vi "Begin (Mark Siekmeier's conflicted copy 2013-04-30).vi"(11 "Image Size":T1=enum."160x120") -> (0 "error out":errorcluster)   [LabVIEW 2012]
doc: "Called before other user functions, this VI is expected to open initial I/O refnums, load in file data, and do all program initialization. Notice that the <B>error out</B> terminal is simply used for data flow. Wiring it to other structures or subVIs ensures that this VI runs first."
uses:
  <vilib>/Rock Robotics/WPI/Camera/WPI_CameraImageSize.ctl
  <vilib>/Rock Robotics/WPI/Camera/WPI_CameraWhite Balance Values.ctl
  <vilib>/Rock Robotics/WPI/Camera/WPI_CameraExposure Values.ctl
  <vilib>/Rock Robotics/WPI/Camera/WPI_CameraFrameRate.ctl
  <vilib>/Rock Robotics/WPI/DriverStation/WPI_DriverStationRobotMode2.ctl
  <vilib>/Rock Robotics/WPI/Joystick/WPI_JoystickDeviceEnum.ctl
  <vilib>/Rock Robotics/SystemInterfaces/Typedef/FPGA_TypedefDigitalModule.ctl
  <vilib>/Rock Robotics/SystemInterfaces/DIO/FPGA_DIOPWMChannel.ctl
  <vilib>/Rock Robotics/WPI/Solenoid/WPI_SolenoidChannel.ctl
  <vilib>/Rock Robotics/SystemInterfaces/Typedef/FPGA_TypedefSolenoidModule.ctl
  <vilib>/Rock Robotics/WPI/Solenoid/WPI_SolenoidValue.ctl
  <vilib>/Rock Robotics/SystemInterfaces/DIO/FPGA_DIOChannel.ctl
  <vilib>/Rock Robotics/WPI/Encoder/WPI_EncoderType.ctl
  <vilib>/Rock Robotics/WPI/SafetyOutput/WPI_SafetyOutputConfigMenu.ctl
  <vilib>/Rock Robotics/SystemInterfaces/DIO/FPGA_DIORelayChannel.ctl
  <vilib>/Rock Robotics/SystemInterfaces/Typedef/FPGA_TypedefAnalogModuleForGyro.ctl
  <vilib>/Rock Robotics/SystemInterfaces/AI/FPGA_AIGyroChannel.ctl
  Robot Global Data.vi
  <vilib>/Rock Robotics/WPI/Solenoid/WPI_SolenoidOpenSingle.vi
  <vilib>/Rock Robotics/WPI/Solenoid/WPI_SolenoidSetEnum.vi
  <vilib>/Rock Robotics/WPI/Counter/WPI_CounterDigitalInputToDigitalSource.vi
  <vilib>/Rock Robotics/WPI/RobotDrive/WPI_RobotDriveOpen2MotorWithTalon.vi
  <vilib>/Rock Robotics/WPI/Solenoid/WPI_SolenoidOpenDouble.vi
  <vilib>/Rock Robotics/WPI/MotorControl/WPI_MotorControlOpen Talon.vi
  <vilib>/Rock Robotics/WPI/Compressor/WPI_CompressorGetSetRefNum.vi
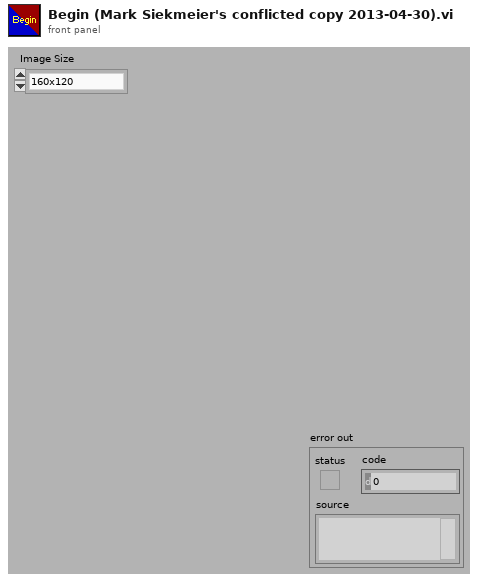
[diagram p1: front panel]
types:
  T1 = typedef "WPI_CameraImageSize.ctl" = enum16{"640x480", "320x240", "160x120"}
  T2 = typedef "FPGA_AIGyroChannel.ctl" = enum8{"AI 1", "AI 2", "Invalid"}
  T3 = typedef "FPGA_TypedefAnalogModuleForGyro.ctl" = enum16{"Analog Module 1"}
  T4 = typedef "WPI_SolenoidChannel.ctl" = enum8{"Solenoid 1", "Solenoid 2", "Solenoid 3", "Solenoid 4", "Solenoid 5", "Solenoid 6", "Solenoid 7", "Solenoid 8", "Invalid"}
  T5 = typedef "WPI_SolenoidValue.ctl" = enum16{"Off", "On", "Forward", "Reverse"}
  T6 = typedef "FPGA_DIOChannel.ctl" = enum8{"DIO 1", "DIO 2", "DIO 3", "DIO 4", "DIO 5", "DIO 6", "DIO 7", "DIO 8", "DIO 9", "DIO 10", "DIO 11", "DIO 12", "DIO 13", "DIO 14", "Invalid"}
  T7 = typedef "FPGA_DIORelayChannel.ctl" = enum8{"Relay 1", "Relay 2", "Relay 3", "Relay 4", "Relay 5", "Relay 6", "Relay 7", "Relay 8", "Invalid"}
  T8 = typedef "FPGA_TypedefDigitalModule.ctl" = enum16{"Digital Module 1", "Digital Module 2"}
  T9 = typedef "WPI_SafetyOutputConfigMenu.ctl" = enum16{"Enable", "Disable"}
  T10 = typedef "FPGA_DIOPWMChannel.ctl" = enum8{"PWM 1", "PWM 2", "PWM 3", "PWM 4", "PWM 5", "PWM 6", "PWM 7", "PWM 8", "PWM 9", "PWM 10", "Invalid"}
  T11 = typedef "WPI_EncoderType.ctl" = enum16{"1x", "2x", "4x"}
  T12 = typedef "FPGA_TypedefSolenoidModule.ctl" = enum16{"Solenoid Module 1", "Solenoid Module 2"}
  T13 = typedef "WPI_JoystickDeviceEnum.ctl" = enum16{"USB 1", "USB 2", "USB 3", "USB 4", "Kinect 1", "Kinect 2"}
  T14 = typedef "WPI_DriverStationRobotMode2.ctl" = enum16{"Autonomous Disabled", "Autonomous Enabled", "Teleop Disabled", "Teleop Enabled", "Timeout", "Finish", "Test Disabled", "Test Enabled"}
  T15 = typedef "WPI_CameraFrameRate.ctl" = u32
  T16 = typedef "WPI_CameraExposure Values.ctl" = enum16{"Auto", "Flicker-free 50 Hz", "Flicker-free 60 Hz", "Hold current"}
  T17 = typedef "WPI_CameraWhite Balance Values.ctl" = enum16{"Auto", "Fixed indoor", "Fixed outdoor 1", "Fixed outdoor 2", "Fixed fluorescent 1", "Fixed fluorescent 2", "Hold current"}
  T18 = typedef "WPI_DigitalInputDevRef.ctl" = cluster{"DevStatus":errorcluster, "DIO Channel":T6, "Digital Module":T8}
  T19 = typedef "WPI_CompressorDevRef.ctl" = cluster{"DevStatus":errorcluster, "DigitalInputDevRef":T18, "RelayDevRef":T20}
  T20 = typedef "WPI_RelayDevRef.ctl" = cluster{"DevStatus":errorcluster, "Relay Channel":T7, "Digital Module":T8, "Relay Direction":T21}
  T21 = typedef "WPI_RelayDirection.ctl" = enum16{"Both directions", "Forward only", "Reverse only"}
  T22 = typedef "FPGA_CounterEncoderSourceConvertionLVSourceType.ctl" = cluster{"DevStatus":errorcluster, "AnalogTriggerMode?":bool, "DigitalMode":cluster{"Digital Module":T8, "DIO Channel":T23}, "AnalogTriggerMode":cluster{"AnalogTriggerIndex":T24, "OutputType":T25}}
  T23 = typedef "FPGA_DIODigitalSourceChannel.ctl" = enum8{"DIO 1", "DIO 2", "DIO 3", "DIO 4", "DIO 5", "DIO 6", "DIO 7", "DIO 8", "DIO 9", "DIO 10", "DIO 11", "DIO 12", "DIO 13", "DIO 14", "Disabled"}
  T24 = typedef "FPGA_AnalogTriggerIndex.ctl" = enum8{"Trig 0", "Trig 1", "Trig 2", "Trig 3", "Trig 4", "Trig 5", "Trig 6", "Trig 7", "Invalid"}
  T25 = typedef "FPGA_AnalogTriggerOutType.ctl" = enum16{"InWindow", "TriggerState", "Rising", "Falling"}
  T26 = typedef "WPI_JoystickDevRef.ctl" = cluster{"Device":T13}
  T27 = typedef "WPI_CameraDevRef.ctl" = cluster{"Camera Address":string, "CameraStatus":errorcluster, "Acquire Image Notifier":refnum<notifier>}
  T28 = typedef "WPI_RobotDriveDevRef.ctl" = cluster{"DevStatus":errorcluster, "Motors[]":T29[], "Square Inputs":bool, "Max Output":dbl, "Isochronous":bool}
  T29 = typedef "WPI_MotorControlDeviceRef.ctl" = cluster{"DeviceStatus":errorcluster, "Type":enum16{"PWM", "CAN"}, "PWM":cluster{"Digital Module":T8, "PWM Channel":T10, "DeadBand":T30}, "CAN":cluster{"Device Number":u8, "Control Mode":T31, "Semaphore":T32, "Max Vout":dbl}, "Invert":bool, "TransformRef":T33, "InvTransformRef":T33}
  T30 = typedef "WPI_PWMDeadband.ctl" = cluster{"Name":string, "maxPositivePwm":i32, "minPositivePwm":i32, "centerPwm":i32, "maxNegativePwm":i32, "minNegativePwm":i32, "angularRange":u16}
  T31 = typedef "WPI_CANJaguar_ControlMode.ctl" = enum8{"Percent VBus", "Current", "Speed", "Position", "Voltage"}
  T32 = typedef "Semaphore RefNum" = refnum<k1>
  T33 = typedef "WPI_PWMTransform_ConPane.ctl" = refnum<vi>
  T34 = typedef "WPI_EncoderDevRef.ctl" = cluster{"DevStatus":errorcluster, "EncoderIndex":T35, "CounterIndex":T36, "DistancePerCount":dbl, "Decoding Type":T11}
  T35 = typedef "FPGA_EncoderIdx.ctl" = enum8{"Enc 0", "Enc 1", "Enc 2", "Enc 3", "Invalid"}
  T36 = typedef "FPGA_CounterCtrSystemIndex.ctl" = enum8{"Ctr 0", "Ctr 1", "Ctr 2", "Ctr 3", "Ctr 4", "Ctr 5", "Ctr 6", "Ctr 7", "Invalid"}
  T37 = typedef "WPI_SolenoidDevRef.ctl" = cluster{"DevStatus":errorcluster, "Solenoid Module":T12, "Forward Solenoid Channel":T4, "Reverse Solenoid Channel":T4}
  T38 = typedef "WPI_GyroDevRef.ctl" = cluster{"DevStatus":errorcluster, "Analog Module":T39, "Analog Channel":T40, "Offset":dbl, "Gain (VoltsPerDegree/Second)":dbl}
  T39 = typedef "FPGA_TypedefAnalogModule.ctl" = enum16{"Analog Module 1", "Analog Module 2"}
  T40 = typedef "FPGA_AIChannel.ctl" = enum8{"AI 1", "AI 2", "AI 3", "AI 4", "AI 5", "AI 6", "AI 7", "AI 8", "Invalid"}
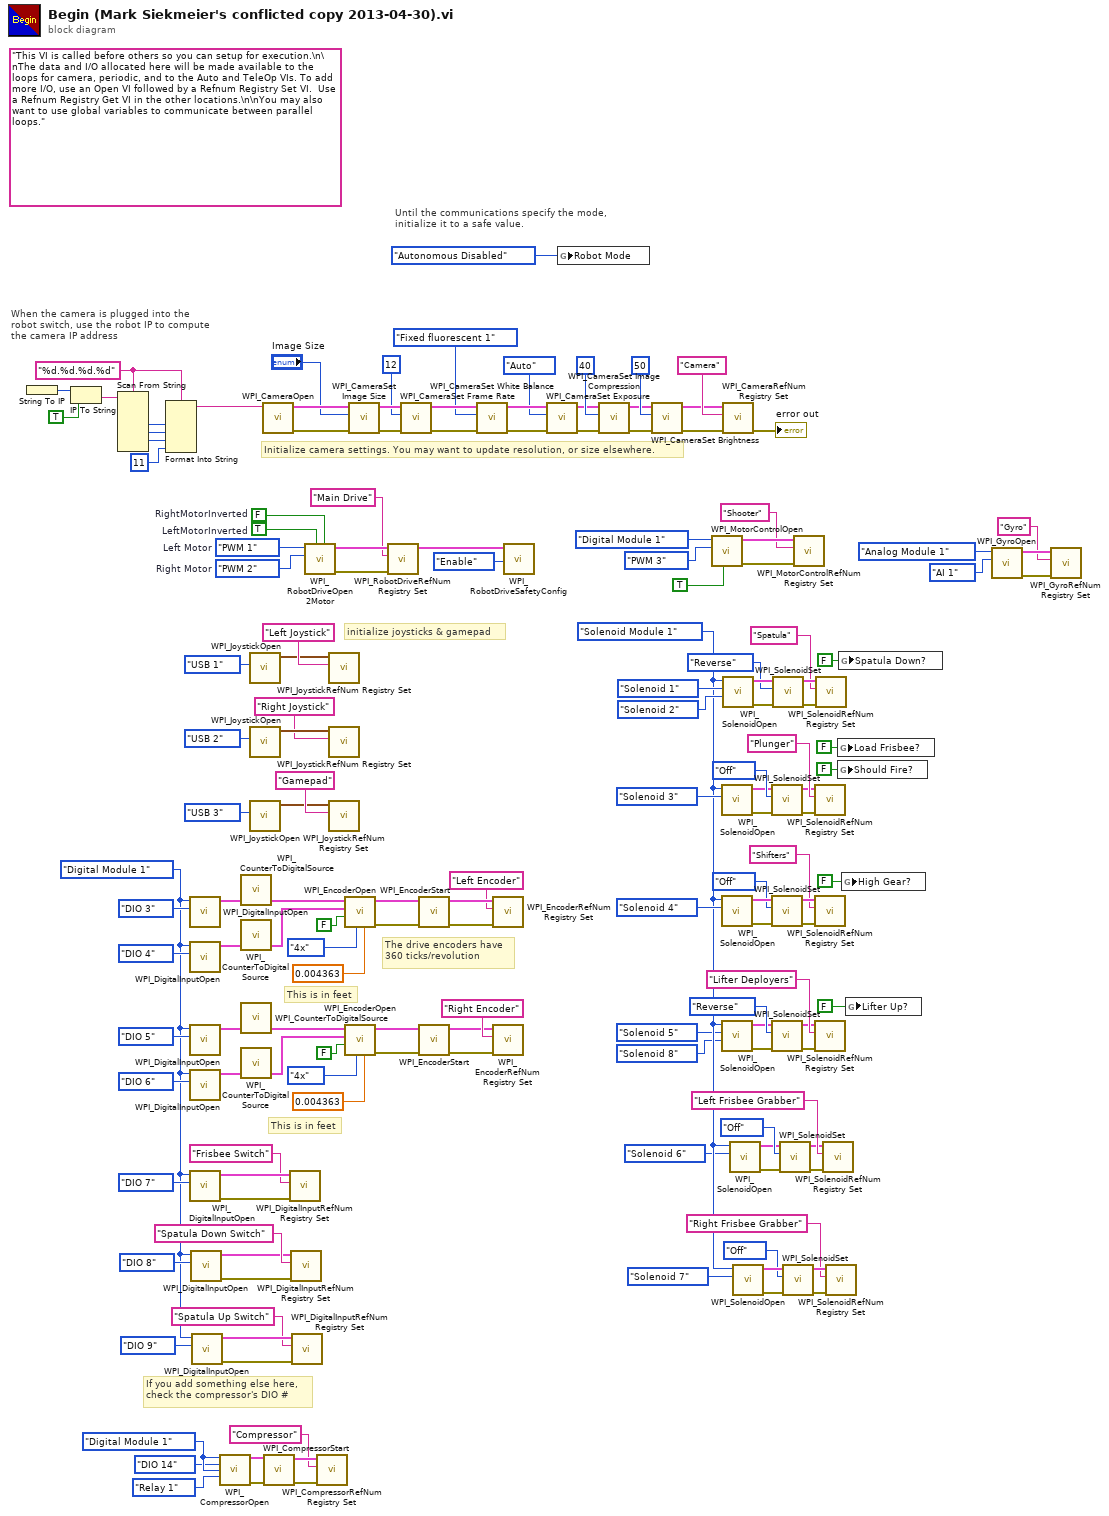
[diagram p0: block diagram]
diagram:
  w47 = FPGA_TypedefDigitalModule."Digital Module 1" ("Pressure Switch Digital Module (Module 1)")
  w65 = FPGA_DIOPWMChannel."PWM 2"  # Right Motor
  w66 = FPGA_DIOPWMChannel."PWM 1"  # Left Motor
  w70 = TRUE  # LeftMotorInverted
  w71 = FALSE  # RightMotorInverted
  w29 = FPGA_TypedefSolenoidModule."Solenoid Module 1" ("Solenoid Module (Module 1)")
  w31 = FPGA_TypedefDigitalModule."Digital Module 1" ("Digital Module (Module 1)")
  w132 = "%d.%d.%d.%d" ("format string")
  (unwired) "This VI is called before others so you can setup for execution.\n\nThe data and I/O allocated here will be made available to the loops for camera, periodic, and to the Auto and TeleOp VIs. To add more I/O, use an Open VI followed by a Refnum Registry Set VI.  Use a Refnum Registry Get VI in the other locations.\n\nYou may also want to use global variables to communicate between parallel loops."
  # "If you add something else here,\ncheck the compressor's DIO #"
  # "The drive encoders have\n360 ticks/revolution"
  # "This is in feet"
  # "This is in feet"
  # "initialize joysticks & gamepad"
  # "Until the communications specify the mode,\ninitialize it to a safe value."
  # "When the camera is plugged into the\nrobot switch, use the robot IP to compute\nthe camera IP address"
  # "Initialize camera settings. You may want to update resolution, or size elsewhere."
  n1 = String To IP() -> (0:w139:u32)  [unwired: 1 in]
  n2 = IP To String(1:TRUE ("dot notation? (F)"), 2:w139) -> (0:w137:string)
  n3 = Scan From String(format string=w132, input string=w137) -> (output 1=w136:i32, output 2=w135:i32, output 3=w134:i32)  [unwired: 7 in, 3 out]
  n4 = Format Into String(format string=w132, w136, w135, w134, 11 ("Compression")) -> (resulting string=w130:string)  [unwired: 2 in, 1 out]
  n5 = call <vilib>:"WPI_DigitalInputOpen.vi"("DIO Channel"=FPGA_DIOChannel."DIO 3" ("CS Channel"), "Digital Module (Module 1)"=w31) -> ("DigitalInputDevRef"=w93:T18)  [unwired: 1 in, 8 out]
  n6 = call <vilib>:"WPI_DigitalInputOpen.vi"("DIO Channel"=FPGA_DIOChannel."DIO 4" ("Clock Channel"), "Digital Module (Module 1)"=w31) -> ("DigitalInputDevRef"=w94:T18)  [unwired: 1 in, 8 out]
  n7 = call <vilib>:"WPI_DigitalInputOpen.vi"("DIO Channel"=FPGA_DIOChannel."DIO 5" ("CS Channel"), "Digital Module (Module 1)"=w31) -> ("DigitalInputDevRef"=w78:T18)  [unwired: 1 in, 8 out]
  n8 = call <vilib>:"WPI_DigitalInputOpen.vi"("DIO Channel"=FPGA_DIOChannel."DIO 6" ("Clock Channel"), "Digital Module (Module 1)"=w31) -> ("DigitalInputDevRef"=w77:T18)  [unwired: 1 in, 8 out]
  n9 = call <vilib>:"WPI_DigitalInputOpen.vi"("DIO Channel"=FPGA_DIOChannel."DIO 7", "Digital Module (Module 1)"=w31) -> ("error out"=w49:errorcluster, "DigitalInputDevRef"=w50:T18)  [unwired: 8 in]
  n10 = call <vilib>:"WPI_DigitalInputOpen.vi"("DIO Channel"=FPGA_DIOChannel."DIO 8", "Digital Module (Module 1)"=w31) -> ("error out"=w38:errorcluster, "DigitalInputDevRef"=w37:T18)  [unwired: 8 in]
  n11 = call <vilib>:"WPI_DigitalInputOpen.vi"("DIO Channel"=FPGA_DIOChannel."DIO 9", "Digital Module (Module 1)"=w31) -> ("error out"=w33:errorcluster, "DigitalInputDevRef"=w34:T18)  [unwired: 8 in]
  n12 = call <vilib>:"WPI_CompressorOpen.vi"("Pressure Switch Digital Module (Module 1)"=w47, "Pressure Switch DIO Channel"=FPGA_DIOChannel."DIO 14", "Relay Digital Module (Module 1)"=w47, "Relay Channel"=FPGA_DIORelayChannel."Relay 1") -> ("CompressorDevRef"=w43:T19, "error out"=w44:errorcluster)  [unwired: 10 in]
  n13 = call-poly <vilib>:"WPI_CounterToDigitalSource.vi"("DigitalInputDevRef"=w93) -> ("Digital Source"=w90:T22)  [unwired: 6 out]
  n14 = call-poly <vilib>:"WPI_CounterToDigitalSource.vi"("DigitalInputDevRef"=w94) -> ("Digital Source"=w91:T22)  [unwired: 6 out]
  n15 = call-poly <vilib>:"WPI_CounterToDigitalSource.vi"("DigitalInputDevRef"=w78) -> ("Digital Source"=w81:T22)  [unwired: 6 out]
  n16 = call-poly <vilib>:"WPI_CounterToDigitalSource.vi"("DigitalInputDevRef"=w77) -> ("Digital Source"=w80:T22)  [unwired: 6 out]
  n17 = call <vilib>:"WPI_JoystickOpen.vi"("JoystickDevice"=WPI_JoystickDeviceEnum."USB 1") -> ("JoystickDevRef"=w128:T26)  [unwired: 10 in]
  n18 = call <vilib>:"WPI_JoystickOpen.vi"("JoystickDevice"=WPI_JoystickDeviceEnum."USB 2") -> ("JoystickDevRef"=w124:T26)  [unwired: 10 in]
  n19 = call <vilib>:"WPI_JoystickOpen.vi"("JoystickDevice"=WPI_JoystickDeviceEnum."USB 3") -> ("JoystickDevRef"=w121:T26)  [unwired: 10 in]
  n20 = call <vilib>:"WPI_CameraOpen.vi"("Camera Address"=w130) -> ("error out"=w151:errorcluster, "CameraDevRef"=w152:T27)  [unwired: 1 in, 8 out]
  n21 = call <vilib>:"WPI_CompressorStart.vi"("error in (no error)"=w44, "CompressorDevRef"=w43) -> ("error out"=w42:errorcluster, "CompressorDevRef"=w41:T19)  [unwired: 8 in]
  n22 = call <vilib>:"WPI_DigitalInputRefNum Registry Set.vi"("error in (no error)"=w49, "refnum name"="Frisbee Switch", "DigitalInputDevRef"=w50) -> ()  [unwired: 7 in, 2 out]
  n23 = call <vilib>:"WPI_DigitalInputRefNum Registry Set.vi"("error in (no error)"=w38, "refnum name"="Spatula Down Switch", "DigitalInputDevRef"=w37) -> ()  [unwired: 7 in, 2 out]
  n24 = call <vilib>:"WPI_DigitalInputRefNum Registry Set.vi"("error in (no error)"=w33, "refnum name"="Spatula Up Switch", "DigitalInputDevRef"=w34) -> ()  [unwired: 7 in, 2 out]
  n25 = call-poly <vilib>:"WPI_RobotDriveOpen2Motor.vi"("Right Motor Inverted"=w71, "Left Motor Inverted"=w70, "Right Motor"=w65, "Left Motor"=w66) -> ("error out"=w67:errorcluster, "RobotDriveDevRef"=w69:T28)  [unwired: 1 in, 5 out]
  n26 = call <vilib>:"WPI_CompressorRefNum Registry Set.vi"("error in (no error)"=w42, "refnum name"="Compressor", "CompressorDevRef"=w41) -> ()  [unwired: 7 in, 2 out]
  n27 = call <vilib>:"WPI_JoystickRefNum Registry Set.vi"("refnum name"="Left Joystick", "JoystickDevRef"=w128) -> ()  [unwired: 8 in, 2 out]
  n28 = call <vilib>:"WPI_JoystickRefNum Registry Set.vi"("refnum name"="Right Joystick", "JoystickDevRef"=w124) -> ()  [unwired: 8 in, 2 out]
  n29 = call <vilib>:"WPI_JoystickRefNum Registry Set.vi"("refnum name"="Gamepad", "JoystickDevRef"=w121) -> ()  [unwired: 8 in, 2 out]
  n30 = call <vilib>:"WPI_EncoderOpen.vi"("DistancePerCount"=0.004363, "Decoding Type"=WPI_EncoderType."4x", "Invert Direction (False)"=FALSE, "BSource"=w91, "ASource"=w90) -> ("error out"=w96:errorcluster, "EncoderDevRef"=w95:T34)  [unwired: 5 in]
  n31 = call <vilib>:"WPI_EncoderOpen.vi"("DistancePerCount"=0.004363, "Decoding Type"=WPI_EncoderType."4x", "Invert Direction (False)"=FALSE, "BSource"=w80, "ASource"=w81) -> ("error out"=w75:errorcluster, "EncoderDevRef"=w76:T34)  [unwired: 5 in]
  n32 = call <vilib>:"WPI_CameraSet Image Size.vi"("error in (no error)"=w151, "Image Size"="Image Size", "CameraDevRef"=w152) -> ("error out"=w150:errorcluster, "CameraDevRef Out"=w153:T27)  [unwired: 7 out]
  n33 = call <vilib>:"WPI_RobotDriveRefNum Registry Set.vi"("error in (no error)"=w67, "refnum name"="Main Drive", "RobotDriveDevRef"=w69) -> ("RobotDriveDevRef"=w64:T28)  [unwired: 8 out]
  n34 = call <vilib>:"WPI_CameraSet Frame Rate.vi"("error in (no error)"=w150, "Frame Rate (fps)"=T15 12, "CameraDevRef"=w153) -> ("error out"=w149:errorcluster, "CameraDevRef Out"=w155:T27)  [unwired: 7 out]
  n35 = call <vilib>:"WPI_EncoderStart.vi"("error in (no error)"=w96, "EncoderDevRef"=w95) -> ("error out"=w97:errorcluster, "EncoderDevRef"=w98:T34)  [unwired: 8 in]
  n36 = call <vilib>:"WPI_EncoderStart.vi"("error in (no error)"=w75, "EncoderDevRef"=w76) -> ("error out"=w74:errorcluster, "EncoderDevRef"=w73:T34)  [unwired: 8 in]
  n37 = call <vilib>:"WPI_CameraSet White Balance.vi"("error in (no error)"=w149, "White Balance"=WPI_CameraWhite_Balance_Values."Fixed fluorescent 1", "CameraDevRef"=w155) -> ("error out"=w148:errorcluster, "CameraDevRef Out"=w154:T27)  [unwired: 7 out]
  n38 = call <vilib>:"WPI_EncoderRefNum Registry Set.vi"("error in (no error)"=w97, "refnum name"="Left Encoder", "EncoderDevRef"=w98) -> ()  [unwired: 7 in, 2 out]
  n39 = call <vilib>:"WPI_EncoderRefNum Registry Set.vi"("error in (no error)"=w74, "refnum name"="Right Encoder", "EncoderDevRef"=w73) -> ()  [unwired: 7 in, 2 out]
  n40 = call <vilib>:"WPI_RobotDriveSafetyConfig.vi"("mode"=WPI_SafetyOutputConfigMenu."Enable", "RobotDriveDevRef"=w64) -> ()  [unwired: 8 in, 2 out]
  n41 = call <vilib>:"WPI_CameraSet Exposure.vi"("error in (no error)"=w148, "Exposure"=WPI_CameraExposure_Values."Auto", "CameraDevRef"=w154) -> ("error out"=w147:errorcluster, "CameraDevRef Out"=w157:T27)  [unwired: 7 out]
  n42 = global write "Robot Global Data.vi" "Robot Mode"(WPI_DriverStationRobotMode2."Autonomous Disabled" ("Robot Mode")) -> ()
  n43 = call <vilib>:"WPI_CameraSet Image Compression.vi"("error in (no error)"=w147, "Compression"=40, "CameraDevRef"=w157) -> ("error out"=w146:errorcluster, "CameraDevRef Out"=w156:T27)  [unwired: 7 out]
  n44 = call <vilib>:"WPI_CameraSet Brightness.vi"("error in (no error)"=w146, "Brightness"=50, "CameraDevRef"=w156) -> ("error out"=w144:errorcluster, "CameraDevRef Out"=w145:T27)  [unwired: 7 out]
  n45 = call-poly <vilib>:"WPI_MotorControlOpen.vi"("Invert"=TRUE, "PWM Channel"=FPGA_DIOPWMChannel."PWM 3", "Digital Module (Module 1)"=FPGA_TypedefDigitalModule."Digital Module 1") -> ("error out"=w116:errorcluster, "MotorControlDeviceRef"=w117:T29)  [unwired: 7 in]
  n46 = call-poly <vilib>:"WPI_SolenoidOpen.vi"("Solenoid Channel"=WPI_SolenoidChannel."Solenoid 3", "Solenoid Module (Module 1)"=w29) -> ("error out"=w104:errorcluster, "SolenoidDevRef"=w103:T37)  [unwired: 8 in]
  n47 = call-poly <vilib>:"WPI_SolenoidOpen.vi"("Solenoid Channel"=WPI_SolenoidChannel."Solenoid 4", "Solenoid Module (Module 1)"=w29) -> ("error out"=w59:errorcluster, "SolenoidDevRef"=w60:T37)  [unwired: 8 in]
  n48 = call-poly <vilib>:"WPI_SolenoidOpen.vi"("Reverse Solenoid Channel"=WPI_SolenoidChannel."Solenoid 8", "Forward Solenoid Channel"=WPI_SolenoidChannel."Solenoid 5" ("Solenoid Channel"), "Solenoid Module (Module 1)"=w29) -> ("error out"=w10:errorcluster, "SolenoidDevRef"=w9:T37)  [unwired: 7 in]
  n49 = call <vilib>:"WPI_CameraRefNum Registry Set.vi"("error in (no error)"=w144, "refnum name"="Camera", "CameraDevRef"=w145) -> ("error out"=→"error out":errorcluster)  [unwired: 8 out]
  n50 = call-poly <vilib>:"WPI_SolenoidOpen.vi"("Reverse Solenoid Channel"=WPI_SolenoidChannel."Solenoid 2", "Forward Solenoid Channel"=WPI_SolenoidChannel."Solenoid 1" ("Solenoid Channel"), "Solenoid Module (Module 1)"=w29) -> ("error out"=w112:errorcluster, "SolenoidDevRef"=w113:T37)  [unwired: 7 in]
  n51 = call-poly <vilib>:"WPI_SolenoidOpen.vi"("Solenoid Channel"=WPI_SolenoidChannel."Solenoid 6", "Solenoid Module (Module 1)"=w29) -> ("error out"=w24:errorcluster, "SolenoidDevRef"=w23:T37)  [unwired: 8 in]
  n52 = call-poly <vilib>:"WPI_SolenoidOpen.vi"("Solenoid Channel"=WPI_SolenoidChannel."Solenoid 7", "Solenoid Module (Module 1)"=w29) -> ("error out"=w19:errorcluster, "SolenoidDevRef"=w20:T37)  [unwired: 8 in]
  n53 = call-poly <vilib>:"WPI_SolenoidSet.vi"("error in (no error)"=w104, "Value"=WPI_SolenoidValue."Off", "SolenoidDevRef"=w103) -> ("error out"=w105:errorcluster, "SolenoidDevRef"=w106:T37)  [unwired: 7 in]
  n54 = call-poly <vilib>:"WPI_SolenoidSet.vi"("error in (no error)"=w59, "Value"=WPI_SolenoidValue."Off", "SolenoidDevRef"=w60) -> ("error out"=w58:errorcluster, "SolenoidDevRef"=w57:T37)  [unwired: 7 in]
  n55 = call-poly <vilib>:"WPI_SolenoidSet.vi"("error in (no error)"=w10, "Value"=WPI_SolenoidValue."Reverse", "SolenoidDevRef"=w9) -> ("error out"=w11:errorcluster, "SolenoidDevRef"=w12:T37)  [unwired: 7 in]
  n56 = call-poly <vilib>:"WPI_SolenoidSet.vi"("error in (no error)"=w112, "Value"=WPI_SolenoidValue."Reverse", "SolenoidDevRef"=w113) -> ("error out"=w111:errorcluster, "SolenoidDevRef"=w110:T37)  [unwired: 7 in]
  n57 = call-poly <vilib>:"WPI_SolenoidSet.vi"("error in (no error)"=w24, "Value"=WPI_SolenoidValue."Off", "SolenoidDevRef"=w23) -> ("error out"=w25:errorcluster, "SolenoidDevRef"=w26:T37)  [unwired: 7 in]
  n58 = call-poly <vilib>:"WPI_SolenoidSet.vi"("error in (no error)"=w19, "Value"=WPI_SolenoidValue."Off", "SolenoidDevRef"=w20) -> ("error out"=w18:errorcluster, "SolenoidDevRef"=w17:T37)  [unwired: 7 in]
  n59 = call <vilib>:"WPI_MotorControlRefNum Registry Set.vi"("error in (no error)"=w116, "refnum name"="Shooter", "MotorControlDevRef"=w117) -> ()  [unwired: 7 in, 2 out]
  n60 = call <vilib>:"WPI_SolenoidRefNum Registry Set.vi"("error in (no error)"=w105, "refnum name"="Plunger", "SolenoidDevRef"=w106) -> ()  [unwired: 7 in, 2 out]
  n61 = call <vilib>:"WPI_SolenoidRefNum Registry Set.vi"("error in (no error)"=w58, "refnum name"="Shifters", "SolenoidDevRef"=w57) -> ()  [unwired: 7 in, 2 out]
  n62 = call <vilib>:"WPI_SolenoidRefNum Registry Set.vi"("error in (no error)"=w11, "refnum name"="Lifter Deployers", "SolenoidDevRef"=w12) -> ()  [unwired: 7 in, 2 out]
  n63 = call <vilib>:"WPI_SolenoidRefNum Registry Set.vi"("error in (no error)"=w111, "refnum name"="Spatula", "SolenoidDevRef"=w110) -> ()  [unwired: 7 in, 2 out]
  n64 = call <vilib>:"WPI_SolenoidRefNum Registry Set.vi"("error in (no error)"=w25, "refnum name"="Left Frisbee Grabber", "SolenoidDevRef"=w26) -> ()  [unwired: 7 in, 2 out]
  n65 = call <vilib>:"WPI_SolenoidRefNum Registry Set.vi"("error in (no error)"=w18, "refnum name"="Right Frisbee Grabber", "SolenoidDevRef"=w17) -> ()  [unwired: 7 in, 2 out]
  n66 = global write "Robot Global Data.vi" "Load Frisbee?"(FALSE ("High Gear?")) -> ()
  n67 = global write "Robot Global Data.vi" "Should Fire?"(FALSE ("High Gear?")) -> ()
  n68 = global write "Robot Global Data.vi" "Spatula Down?"(FALSE ("High Gear?")) -> ()
  n69 = global write "Robot Global Data.vi" "High Gear?"(FALSE ("High Gear?")) -> ()
  n70 = global write "Robot Global Data.vi" "Lifter Up?"(FALSE ("High Gear?")) -> ()
  n71 = call <vilib>:"WPI_GyroOpen.vi"("Analog Channel"=FPGA_AIGyroChannel."AI 1", "Analog Module (Module 1)"=FPGA_TypedefAnalogModuleForGyro."Analog Module 1") -> ("error out"=w5:errorcluster, "GyroDevRef"=w4:T38)  [unwired: 7 in, 1 out]
  n72 = call <vilib>:"WPI_GyroRefNum Registry Set.vi"("error in (no error)"=w5, "refnum name"="Gyro", "GyroDevRef"=w4) -> ()  [unwired: 7 in, 2 out]
